vi "R@Isc and R@Voc.vi"(10 "percentage":sgl=0.075, 11 "Current (Amps) vs Voltage (Volts)":cluster{"Array":dbl[], "Array":dbl[]}) -> (1 "Rseries":dbl format="%#.6g", 2 "Rshunt":dbl format="%#.6g", 3 "Current (Amps) vs Voltage (Volts) 2":cluster{"Array":dbl[], "Array":dbl[]}[](graph))   [LabVIEW 2016]
uses:
  <vilib>/Analysis/NI_AALPro.lvlib
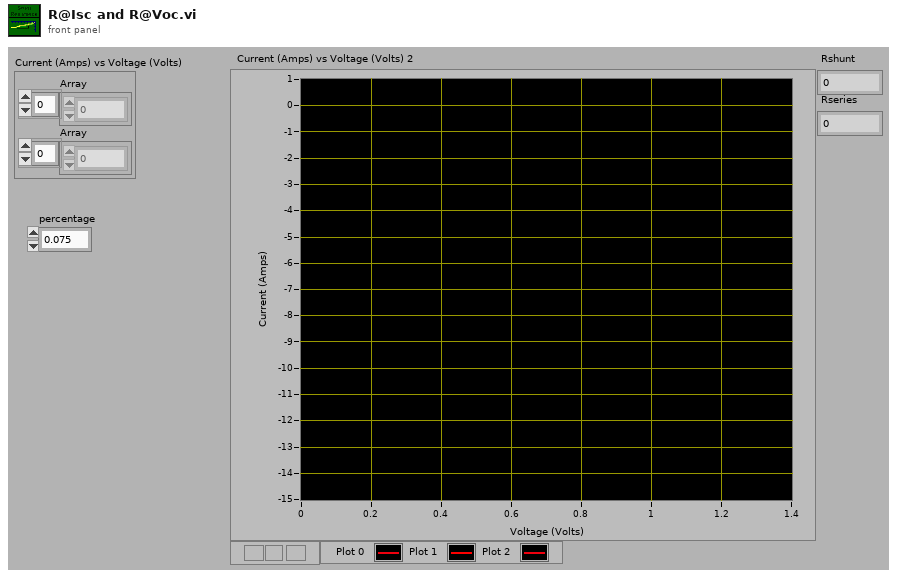
[diagram p1: front panel]
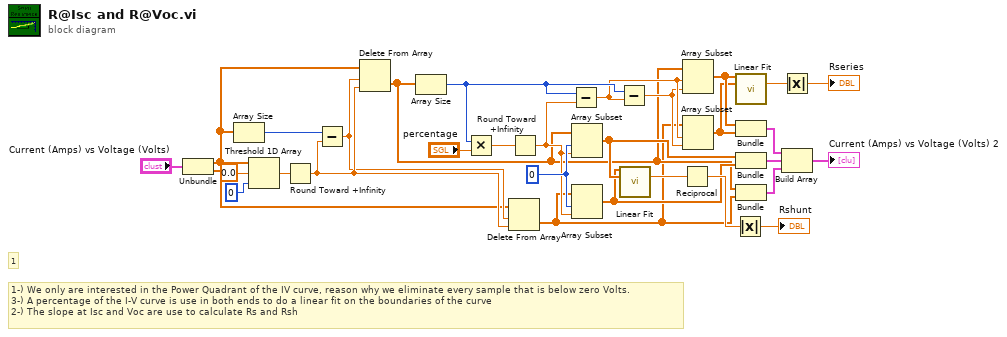
[diagram p0: block diagram]
diagram:
  w13 = 0 ("index")
  # "1"
  # "1-) We only are interested in the Power Quadrant of the IV curve, reason why we eliminate every sample that is below zero Volts.\n3-) A percentage of the I-V curve is use in both ends to do a linear fit on the boundaries of the curve\n2-) The slope at Isc and Voc are use to calculate Rs and Rsh"
  n1 = Unbundle("Current (Amps) vs Voltage (Volts)") -> ("Array"=w27:dbl[], "Array"=w24:dbl[])
  n2 = Array Size(array=w27) -> (size(s)=w12:i32)
  n3 = Threshold 1D Array(1:0 ("start index (0)"), 2:0.0 ("threshold y"), 3:w27) -> (0:w28:dbl)
  n4 = Round Toward +Infinity(x=w28) -> (ceil(x): smallest int >= x=w26:dbl)
  n5 = Subtract(x=w12, y=w26) -> (x-y=w25:dbl)
  n6 = Delete From Array(array=w27, length=w25, index=w26) -> (deleted portion=w6:dbl[])  [unwired: 1 out]
  n7 = Array Size(array=w6) -> (size(s)=w10:i32)
  n8 = Multiply(x=w10, y="percentage") -> (x*y=w19:sgl)
  n9 = Delete From Array(array=w24, length=w25, index=w26) -> (deleted portion=w5:dbl[])  [unwired: 1 out]
  n10 = Round Toward +Infinity(x=w19) -> (ceil(x): smallest int >= x=w11:sgl)
  n11 = Subtract(x=w10, y=w11) -> (x-y=w9:sgl)
  n12 = Array Subset(array=w6, index=w13, length=w11) -> (w17:dbl[])
  n13 = Array Subset(array=w5, index=w13, length=w11) -> (w16:dbl[])
  n14 = Subtract(x=w10, y=w9) -> (x-y=w8:sgl)
  n15 = call <vilib>:"Linear Fit.vi"("Y"=w16, "X"=w17) -> ("slope"=w23:dbl)  [unwired: 4 in, 9 out]
  n16 = Reciprocal(x=w23) -> (1/x=w22:dbl)
  n17 = Array Subset(array=w6, index=w9, length=w8) -> (w3:dbl[])
  n18 = Array Subset(array=w5, index=w9, length=w8) -> (w2:dbl[])
  n19 = Absolute Value(x=w22) -> (abs(x)=→"Rshunt":dbl)
  n20 = call <vilib>:"Linear Fit.vi"("Y"=w3, "X"=w2) -> ("slope"=w1:dbl)  [unwired: 4 in, 9 out]
  n21 = Bundle(w3, w2) -> (w7:cluster{dbl[], dbl[]})  [unwired: 1 out]
  n22 = Bundle(w17, w16) -> (w14:cluster{dbl[], dbl[]})  [unwired: 1 out]
  n23 = Bundle("Array"=w6, "Array"=w5) -> (w15:cluster{"Array":dbl[], "Array":dbl[]})  [unwired: 1 out]
  n24 = Absolute Value(x=w1) -> (abs(x)=→"Rseries":dbl)
  n25 = Build Array(w7, w14, w15) -> (→"Current (Amps) vs Voltage (Volts) 2":cluster{"Array":dbl[], "Array":dbl[]}[])
